vi "Update Boolean.vi"(8 "error in (no error)":errorcluster, 10 "Boolean":bool, 11 "Alternative Example Sink in":refnum<class "Alternative Example Sink.lvclass">) -> (0 "error out":errorcluster, 3 "Alternative Example Sink out":refnum<class "Alternative Example Sink.lvclass">)   [LabVIEW 2016, in "Alternative Example Sink.lvlib" / "Alternative Example Sink.lvclass"]
uses:
  Alternative Example Sink.lvclass
  Alternative Example Sink.lvclass/Alternative Example Sink.ctl
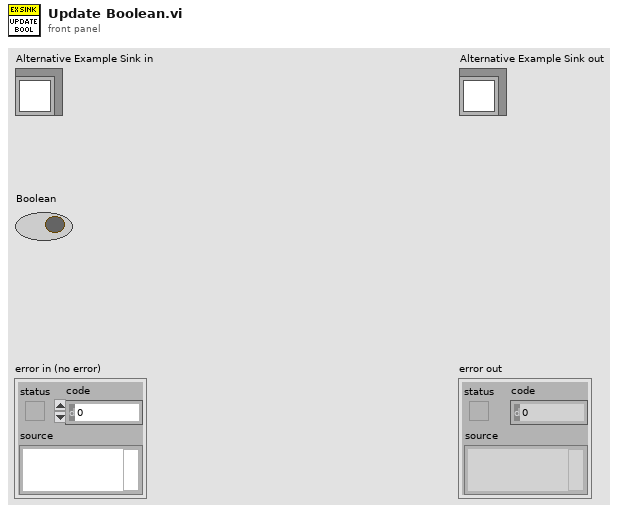
[diagram p1: front panel]
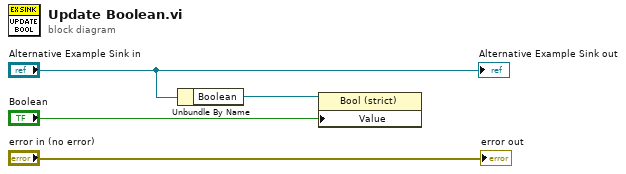
[diagram p0: block diagram]
diagram:
  n1 = Unbundle By Name("Alternative Example Sink in") -> ("Boolean"=w2:refnum<vi>)
  n2 = property class="Bool (strict)"(reference=w2, "Value"="Boolean") -> ()  [unwired: 1 in, 2 out]
  "error out" <- "error in (no error)"
  "Alternative Example Sink out" <- "Alternative Example Sink in"
